vi "Close Child.vi"(8 "error in (no error)":errorcluster, 11 "TCP Client in":refnum<class "TCP Client.lvclass">) -> (0 "error out":errorcluster, 3 "TCP Client out":refnum<class "TCP Client.lvclass">)   [LabVIEW 2020, in "Stream-TCP.lvlib" / "TCP Client.lvclass"]
uses:
  TCP Client.lvclass
  C:/Program Files (x86)/National Instruments/LabVIEW 2020/vi.lib/IlluminatedG/lv-stream/Connection/Connection.lvclass
  Client Command.ctl
  <vilib>/IlluminatedG/lv-stream/Connection/State.ctl
  TCP Client.lvclass/TCP Client.ctl
  Stream-TCP.lvlib
  <vilib>/IlluminatedG/lv-stream/Connection/Connection.lvclass
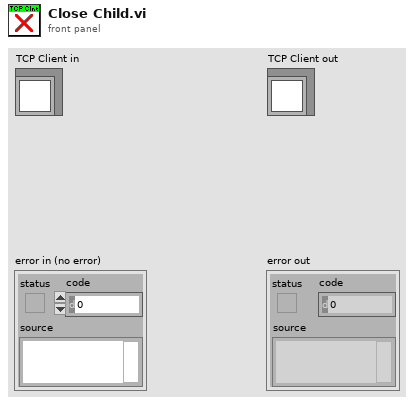
[diagram p1: front panel]
types:
  T1 = typedef "Stream.lvlib/Connection.lvclass/State.ctl" = enum16{"Closed", "Idle", "Connecting", "Connected", "Shutdown"}
  T2 = typedef "Stream-TCP.lvlib/Client Command.ctl" = enum16{"Connect", "Close", "Shutdown", "Reconnect"}
  T3 = typedef "Stream-TCP.lvlib/Client Command Queue.ctl" = refnum<queue>
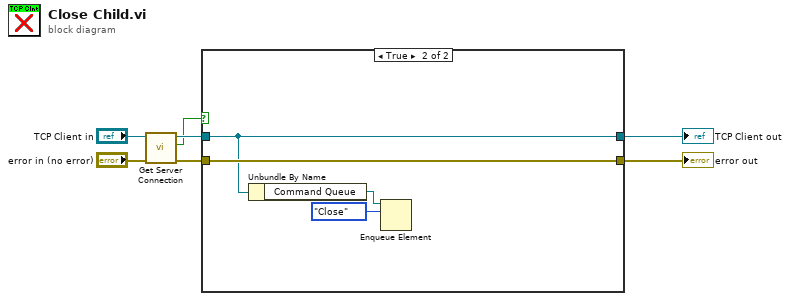
[diagram p0: block diagram]
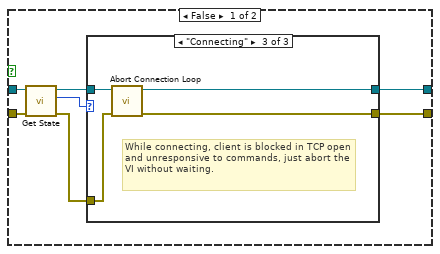
[diagram p2: hidden frame]
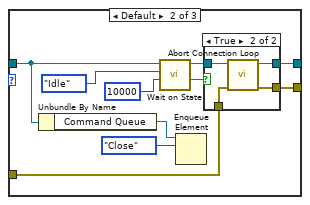
[diagram p4: hidden frame]
diagram:
  n1 = call "Get Server Connection.vi"("error in (no error)"="error in (no error)", "TCP Client in"="TCP Client in") -> ("error out"=w3:errorcluster, "Is Server Connection"=w1:bool, "TCP Client out"=w2:refnum<class "TCP Client.lvclass">)  [unwired: 7 in]
  n2 = case shown="True" w1 {
    tunnel: [w14 w37] -> w7
    tunnel: [w13 w38] -> w6
    tunnel: w3 -> [w9 w38]
    tunnel: w2 -> [w8 w37]
    frame False {
      n3 = call <vilib>:"Get State.vi"("error in (no error)"=w9, "Connection in"=w8) -> ("error out"=w12:errorcluster, "State"=w10:T1, "Connection out"=w11:refnum<class "TCP Client.lvclass">)  [unwired: 7 in]
      n4 = case shown="\"Connecting\"" w10 {
        tunnel: [w16 w24 w34] -> w14
        tunnel: w12 -> [w15 w23 w35]
        tunnel: [w15 w22 w33] -> w13
        tunnel: w11 -> [w16 w21 w36]
        frame "Closed", "Idle" {
        }
        frame Default {
          n5 = Unbundle By Name(w21) -> ("Command Queue"=w26:T3)
          n6 = call <vilib>:"Wait on State.vi"("Timeout ms (-1)"=10000, "State"=State."Idle", "Connection in"=w21) -> ("Timed Out?"=w17:bool, "Connection out"=w18:refnum<class "TCP Client.lvclass">)  [unwired: 6 in, 1 out]
          n7 = Enqueue Element(queue=w26, element=Client_Command."Close") -> ()  [unwired: 2 in, 3 out]
          n8 = case shown="True" w17 {
            tunnel: w18 -> [w28 w32]
            tunnel: [w28 w31] -> w24
            tunnel: w23 -> [w27 w30]
            tunnel: [w27 w29] -> w22
            frame False {
            }
            frame True {
              n9 = call "Abort Connection Loop.vi"("error in (no error)"=w30, "TCP Client in"=w32) -> ("error out"=w29:errorcluster, "TCP Client out"=w31:refnum<class "TCP Client.lvclass">)  [unwired: 8 in]
            }
          }
        }
        frame "Connecting" {
          # "While connecting, client is blocked in TCP open and unresponsive to commands, just abort the VI without waiting."
          n10 = call "Abort Connection Loop.vi"("error in (no error)"=w35, "TCP Client in"=w36) -> ("error out"=w33:errorcluster, "TCP Client out"=w34:refnum<class "TCP Client.lvclass">)  [unwired: 8 in]
        }
      }
    }
    frame True {
      n11 = Unbundle By Name(w37) -> ("Command Queue"=w40:T3)
      n12 = Enqueue Element(queue=w40, element=Client_Command."Close") -> ()  [unwired: 2 in, 3 out]
    }
  }
  "error out" <- w6
  "TCP Client out" <- w7
